vi "KM_messaround V1.vi"() -> ()   [LabVIEW 2016]
panel:
  out "Plot: All 2":cluster{dbl[], dbl[]}(graph)
  in  "N":i32=100
  in  "df 2":dbl=100.0
  in  "freq max 2":dbl=50000.0
  in  "freq min 2":dbl=40000.0
  out "Plot: All":cluster{dbl[], dbl[]}[](graph)=[{[12671.629418564153, 33826.262956804436, 38095.4524796477, 39931.58550466134, 40954.886644874954, 41608.31787374224, 42062.462089613204, 42396.9869830655, 42654.09282963714, 42858.22172100238, 43024.50979540664, 43162.831546920075, 43279.90365252392, 43380.45411679005, 43467.90780314024, 43544.806686718635, 43613.07733690696, 43674.206720122485, 43729.36100318892, 43779.467813457726, 43825.27443094047, 43867.389746861736, 43906.3150381164, 43942.46688852968, 43976.194500421305, 44007.79293629195, 44037.51336571015, 44065.57107980928, 44092.15182185869, 44117.41683369049, 44141.50691295105, 44164.54570127916, 44186.642369379035, 44207.89382536845, 44228.38654352578, 44248.19808872484, 44267.39839540136, 44286.050847404236, 44304.213195521086, 44321.93834209311, 44339.27501640885, 44356.268360095135, 44372.96043821303, 44389.39068899858, 44405.59632299912, 44421.61268062058, 44437.47355572784, 44453.211491855225, 44468.85805673511, 44484.44410019728, 44500.0, 44515.55589980272, 44531.14194326489, 44546.788508144775, 44562.52644427216, 44578.38731937942, 44594.40367700088, 44610.60931100142, 44627.03956178697, 44643.731639904865, 44660.72498359115, 44678.06165790689, 44695.786804478914, 44713.949152595764, 44732.60160459864, 44751.80191127516, 44771.61345647422, 44792.10617463155, 44813.357630620965, 44835.45429872084, 44858.49308704895, 44882.58316630951, 44907.84817814131, 44934.42892019072, 44962.48663428985, 44992.20706370805, 45023.805499578695, 45057.53311147032, 45093.684961883606, 45132.610253138264, 45174.72556905953, 45220.532186542274, 45270.63899681108, 45325.793279877515, 45386.92266309304, 45455.193313281365, 45532.09219685976, 45619.54588320995, 45720.09634747608, 45837.168453079925, 45975.49020459336, 46141.77827899762, 46345.90717036286, 46603.0130169345, 46937.537910386796, 47391.68212625776, 48045.113355125046, 49068.41449533867, 50904.5475203523, 55173.73704319561], [1.7867861029092062e-06, 4.981169044016939e-06, 7.130475296927041e-06, 2.9257331508984305e-06, 2.510807913681395e-06, 2.0809207834550163e-06, 2.4014187118520916e-06, 2.411890426934674e-06, 2.1742789171059614e-06, 2.247745502910839e-06, 2.2141592105407348e-06, 2.226569513729546e-06, 2.3774818297357516e-06, 2.2993414040118902e-06, 2.1121558445415588e-06, 2.0530936064124896e-06, 2.121675856573529e-06, 2.24747478036386e-06, 1.945606021768901e-06, 2.144712914189008e-06, 2.1656259327905262e-06, 1.9663926236744737e-06, 1.752122883402883e-06, 1.8773380244322181e-06, 1.8862551719377669e-06, 1.6503294168233907e-06, 1.8107629374719058e-06, 1.6076381408193275e-06, 1.51850542559986e-06, 1.5579229862230578e-06, 1.288543318486219e-06, 1.3259775681154714e-06, 1.0819164215728348e-06, 9.497489585716396e-07, 8.341516236220823e-07, 3.971917177795927e-07, 1.8343301103831205e-07, -1.837752902056375e-08, -3.33425228167892e-07, -8.176685561251998e-07, -1.7080463904899399e-06, -2.5473226607391914e-06, -3.6708647609780918e-06, -4.474447992693196e-06, -7.239063660913629e-06, -1.008871125370249e-05, -1.4226248018206567e-05, -2.0554700017742062e-05, -3.752039485557242e-05, -6.720037435002469e-05, -0.00011659798571001265, -0.00021204504852284005, -0.0007421766514160975, -0.0009485143391296364, -0.0002584192447894942, -0.0001018744251434476, -4.627993950111265e-05, -2.8504910664511987e-05, -1.925990086172203e-05, -1.3971445626644708e-05, -1.0299887959059592e-05, -7.1575064065682086e-06, -5.82767968858325e-06, -4.551707675681623e-06, -1.2604299149623052e-06, -3.015162826092337e-06, -1.6116614117983256e-06, -1.30904906065693e-06, -7.66156734053056e-07, -1.130729962752735e-06, 1.0638734197523924e-06, -6.478313029527774e-07, 4.3167723834538795e-07, 6.321961814070043e-07, 3.997492706518208e-07, 1.5490815694740424e-08, 1.0911156214235839e-06, 1.0242936641230751e-06, 1.1296536319216856e-06, 8.811154261660182e-07, 1.2531830182366842e-06, 1.398081596607912e-06, 1.4615606671278864e-06, 1.5508537884379647e-06, 1.5221983435149239e-06, 1.7860103098836129e-06, 1.5458311099947898e-06, 1.6948847427874876e-06, 1.548561591366189e-06, 1.5342902197431919e-06, 1.788982294848683e-06, 1.8395292951564845e-06, 1.7672642642682633e-06, 1.6996712843835181e-06, 1.8164451294326104e-06, 1.6964637588764735e-06, 1.7374764358282346e-06, 1.804996666482294e-06, 1.6229667615079487e-06, 1.6199262014483797e-06]}, {[12671.629418564153, 33826.262956804436, 38095.4524796477, 39931.58550466134, 40954.886644874954, 41608.31787374224, 42062.462089613204, 42396.9869830655, 42654.09282963714, 42858.22172100238, 43024.50979540664, 43162.831546920075, 43279.90365252392, 43380.45411679005, 43467.90780314024, 43544.806686718635, 43613.07733690696, 43674.206720122485, 43729.36100318892, 43779.467813457726, 43825.27443094047, 43867.389746861736, 43906.3150381164, 43942.46688852968, 43976.194500421305, 44007.79293629195, 44037.51336571015, 44065.57107980928, 44092.15182185869, 44117.41683369049, 44141.50691295105, 44164.54570127916, 44186.642369379035, 44207.89382536845, 44228.38654352578, 44248.19808872484, 44267.39839540136, 44286.050847404236, 44304.213195521086, 44321.93834209311, 44339.27501640885, 44356.268360095135, 44372.96043821303, 44389.39068899858, 44405.59632299912, 44421.61268062058, 44437.47355572784, 44453.211491855225, 44468.85805673511, 44484.44410019728, 44500.0, 44515.55589980272, 44531.14194326489, 44546.788508144775, 44562.52644427216, 44578.38731937942, 44594.40367700088, 44610.60931100142, 44627.03956178697, 44643.731639904865, 44660.72498359115, 44678.06165790689, 44695.786804478914, 44713.949152595764, 44732.60160459864, 44751.80191127516, 44771.61345647422, 44792.10617463155, 44813.357630620965, 44835.45429872084, 44858.49308704895, 44882.58316630951, 44907.84817814131, 44934.42892019072, 44962.48663428985, 44992.20706370805, 45023.805499578695, 45057.53311147032, 45093.684961883606, 45132.610253138264, 45174.72556905953, 45220.532186542274, 45270.63899681108, 45325.793279877515, 45386.92266309304, 45455.193313281365, 45532.09219685976, 45619.54588320995, 45720.09634747608, 45837.168453079925, 45975.49020459336, 46141.77827899762, 46345.90717036286, 46603.0130169345, 46937.537910386796, 47391.68212625776, 48045.113355125046, 49068.41449533867, 50904.5475203523, 55173.73704319561], [0.0007966200874007219, 0.0007977919093490139, 0.0008006182121907198, 0.000801493824316476, 0.000801907898029911, 0.0008033309731613956, 0.0008041281204714157, 0.0008049298712573447, 0.000805675202033351, 0.0008068129976160579, 0.0008076334425690525, 0.0008085150034351802, 0.0008094711704262918, 0.0008106318414679131, 0.0008114706067046321, 0.0008125010703383446, 0.0008139035103294367, 0.00081473942463114, 0.0008159483635947111, 0.0008167654948798785, 0.0008183953656626397, 0.0008195586175130348, 0.0008207247841030989, 0.000821865060315311, 0.0008237545224164506, 0.0008251803793115513, 0.0008266655787082107, 0.0008282489555769015, 0.0008302678958047276, 0.0008319671258232857, 0.0008339681113024564, 0.0008359754349092745, 0.0008389258926614182, 0.0008413524527918291, 0.0008439753702515234, 0.0008469600600945358, 0.0008513400616966437, 0.0008549359661273672, 0.0008591276974909012, 0.0008635772056161829, 0.0008704108121733616, 0.0008764422356233635, 0.0008842296668849478, 0.0008924014758625232, 0.0009068485064660632, 0.000921206545678709, 0.0009376155622107205, 0.0009602351602920117, 0.0010050215360238514, 0.001057573933276468, 0.0011170165628214693, 0.0012246148574828373, 0.0012097081954509082, 0.0003815291900482268, 0.0002831114535453973, 0.0004515795113362355, 0.0005635076553534257, 0.0006111511038700257, 0.0006405288627858329, 0.000663881432025881, 0.000681161402347664, 0.0006988421046510184, 0.0007088795426047166, 0.0007177588939033982, 0.0007266999216420724, 0.0007323628917056363, 0.0007376497446687229, 0.0007423892020085652, 0.0007469836904060264, 0.0007510747994463339, 0.0007553912814291702, 0.00075679631534775, 0.0007605283789082798, 0.0007628078895875729, 0.0007647694944770409, 0.0007675241530415401, 0.000769432353436328, 0.0007714064705971689, 0.0007727018034463155, 0.0007741631822403668, 0.0007763493377675348, 0.0007776395322550355, 0.0007788385278299043, 0.0007804449781308258, 0.000781793800149987, 0.000783092168788752, 0.0007841220832254033, 0.0007852018106106987, 0.0007862779190199201, 0.0007873357065491119, 0.0007884887472697837, 0.0007897184537534949, 0.0007905263655644359, 0.0007913417735276632, 0.0007923256758648212, 0.0007936705282804686, 0.0007943361837412446, 0.0007951118461760056, 0.0007959176381220687, 0.0007964802645719539]}]
  in  "Error In":errorcluster
  in  "gamma":dbl=1000.0
  in  "omega0":dbl=44500.0
  out "Error Out":errorcluster
  in  "Address":string="DEV3523"
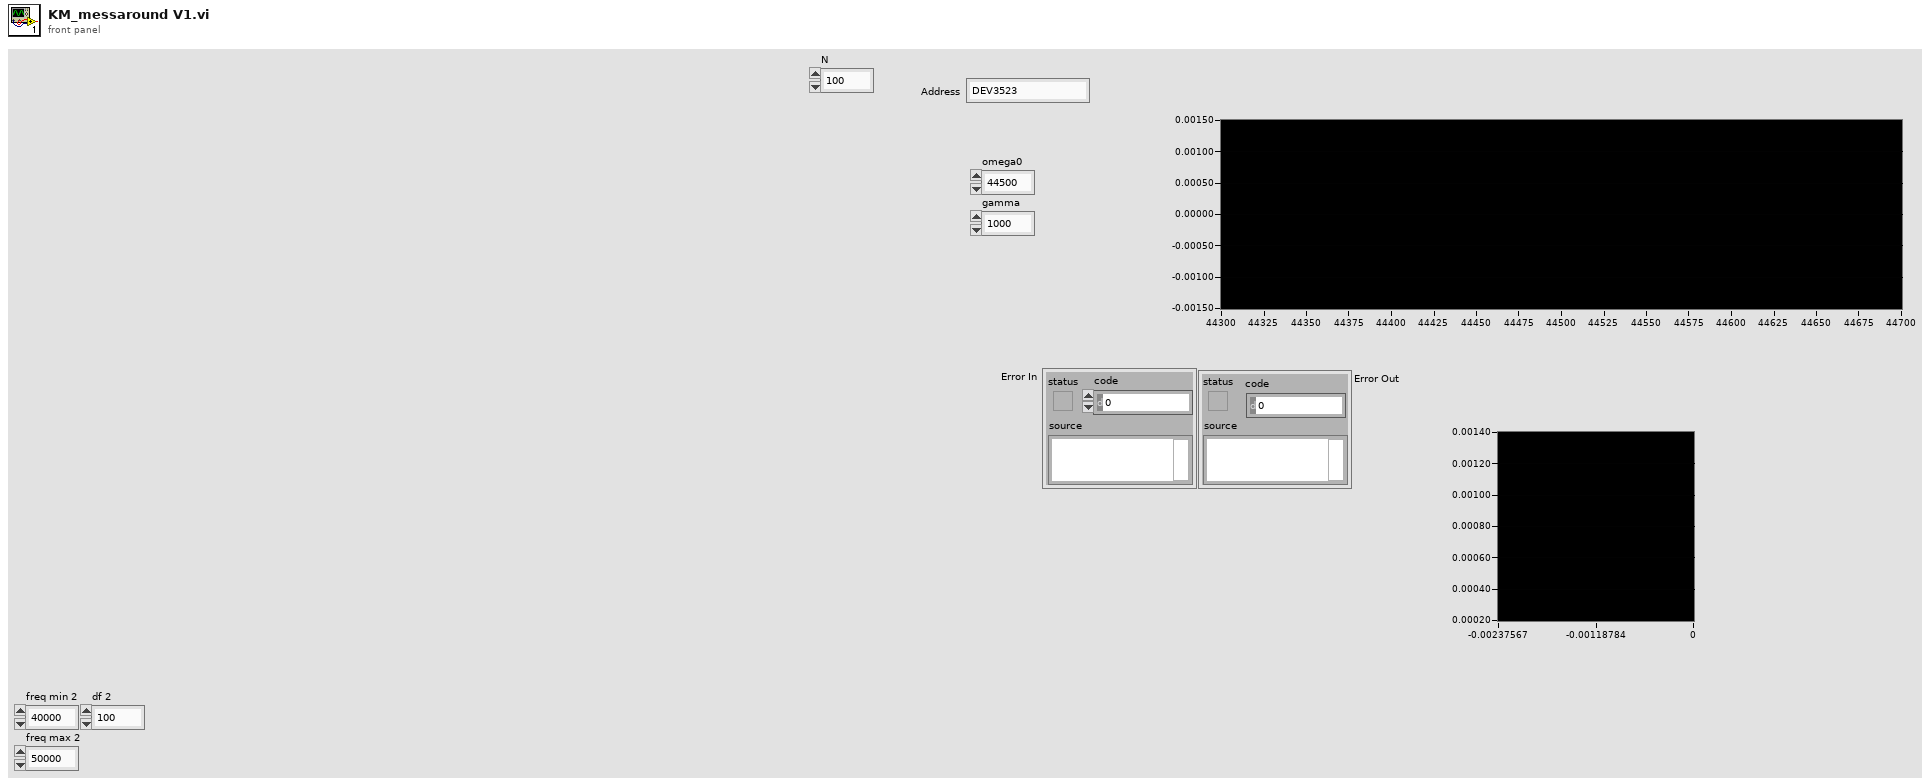
[diagram p1: front panel]
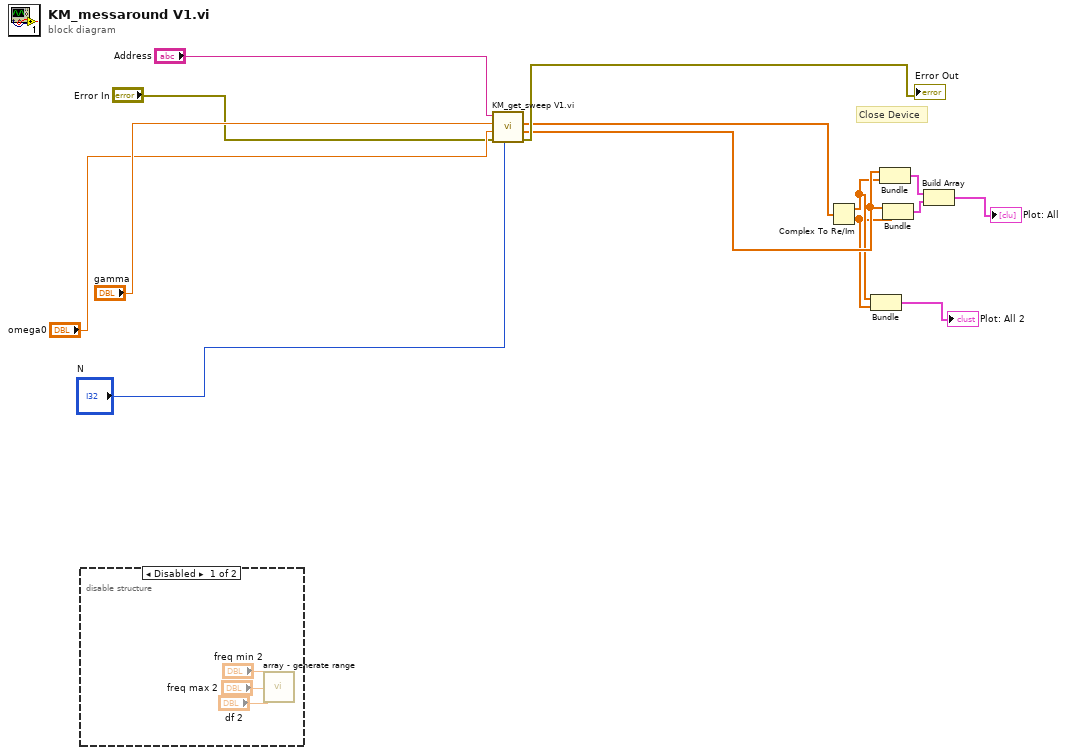
[diagram p0: block diagram]
diagram:
  # "Close Device"
  n1 = disable-structure shown="Disabled" {
    frame Disabled {
      n2 = call "array - generate range.vi"("df"="df 2", "freq max"="freq max 2", "freq min"="freq min 2") -> ()  [unwired: 7 in, 2 out]
    }
    frame Enabled {
    }
  }
  n3 = call "KM_get_sweep V1.vi.vi"("N"="N", "Error In"="Error In", "omega0 (Hz)"="omega0", "gamma (Hz)"="gamma", "Address"="Address") -> ("Error Out"=→"Error Out":errorcluster, "freq out (Hz)"=w4:dbl[], "voltage out (V)"=w5:cdb[])  [unwired: 4 in]
  n4 = Complex To Re/Im(x + iy=w5) -> (x=w3:dbl[], y=w2:dbl[])
  n5 = Bundle(w3, w2) -> (→"Plot: All 2":cluster{dbl[], dbl[]})  [unwired: 1 in]
  n6 = Bundle("freq out (Hz)"=w4, w3) -> (w14:cluster{"freq out (Hz)":dbl[], dbl[]})  [unwired: 1 in]
  n7 = Bundle("freq out (Hz)"=w4, w2) -> (w13:cluster{"freq out (Hz)":dbl[], dbl[]})  [unwired: 1 in]
  n8 = Build Array(w14, w13) -> (→"Plot: All":cluster{"freq out (Hz)":dbl[], dbl[]}[])
